vi "live view D06.vi"() -> ()   [LabVIEW 2019, in "D06.lvlib"]
uses:
  D06.lvlib
  <vilib>/userDefined/High Color/IMAQdx.ctl
  <vilib>/vision/Image Controls.llb/IMAQ Image.ctl
  <vilib>/measure/mamon.llb/Trigger Detection for 1 Channel.vi
  <vilib>/measure/NI_MAPro.lvlib
  Calibration Lib.lvlib
  database.lvlib
  <vilib>/vision/driver/NI_Vision_Acquisition_Software.lvlib
panel:
  out "error out":errorcluster
  in  "snapshot":bool
  out "projector D06 error":errorcluster
  in  "Path":path
  in  "Verify Calibration D06":bool caption="capture grab"
  out "factor":sgl
  out "transform matrix":sgl[](array[numeric])
  in  "Method 2 save D06":bool caption="capture grab"
  in  "Method 1 Save D06":bool caption="Saving txt"
  in  "Close":bool
  out "Average Result":string="Average Result"
  out ">18  A":dbl(slide)=1.0 caption=">18 mm" scale=0.0..100.0
  out "16-18  A":dbl(slide)=1.0 caption="16-18 mm" scale=0.0..100.0
  out "14-16  A":dbl(slide)=1.0 caption="14-16 mm" scale=0.0..100.0
  out "12.5-14 A":dbl(slide)=1.0 caption="12.5-14 mm" scale=0.0..100.0
  out "10-12.5  A":dbl(slide)=1.0 caption="10-12.5 mm" scale=0.0..100.0 scale format="%#_4f"
  out "8-10  A":dbl(slide)=1.0 caption="8-10 mm" scale=0.0..100.0
  out "6.3-8  A":dbl(slide)=1.0 caption="6.3-8 mm" scale=0.0..100.0
  out "<6.3  A":dbl(slide)=1.0 caption="<6.3 mm" scale=0.0..100.0
  out "Live Result":string="Live Result"
  out ">18  L":dbl(slide)=1.0 caption=">18 mm" scale=0.0..100.0
  out "Live View":T1(plugin-control) caption="Disc 26"
  out "16-18  L":dbl(slide)=1.0 caption="16-18 mm" scale=0.0..100.0
  out "14-16  L":dbl(slide)=1.0 caption="14-16 mm" scale=0.0..100.0
  out "12.5-14 L":dbl(slide)=1.0 caption="12.5-14 mm" scale=0.0..100.0
  out "10-12.5  L":dbl(slide)=1.0 caption="10-12.5 mm" scale=0.0..100.0 scale format="%#_4f"
  out "8-10  L":dbl(slide)=1.0 caption="8-10 mm" scale=0.0..100.0
  out "6.3-8  L":dbl(slide)=1.0 caption="6.3-8 mm" scale=0.0..100.0
  out "<6.3  L":dbl(slide)=1.0 caption="<6.3 mm" scale=0.0..100.0
  out "disc name":string="Live Info Disc 06"
  out "dsgs":string="DSGS"
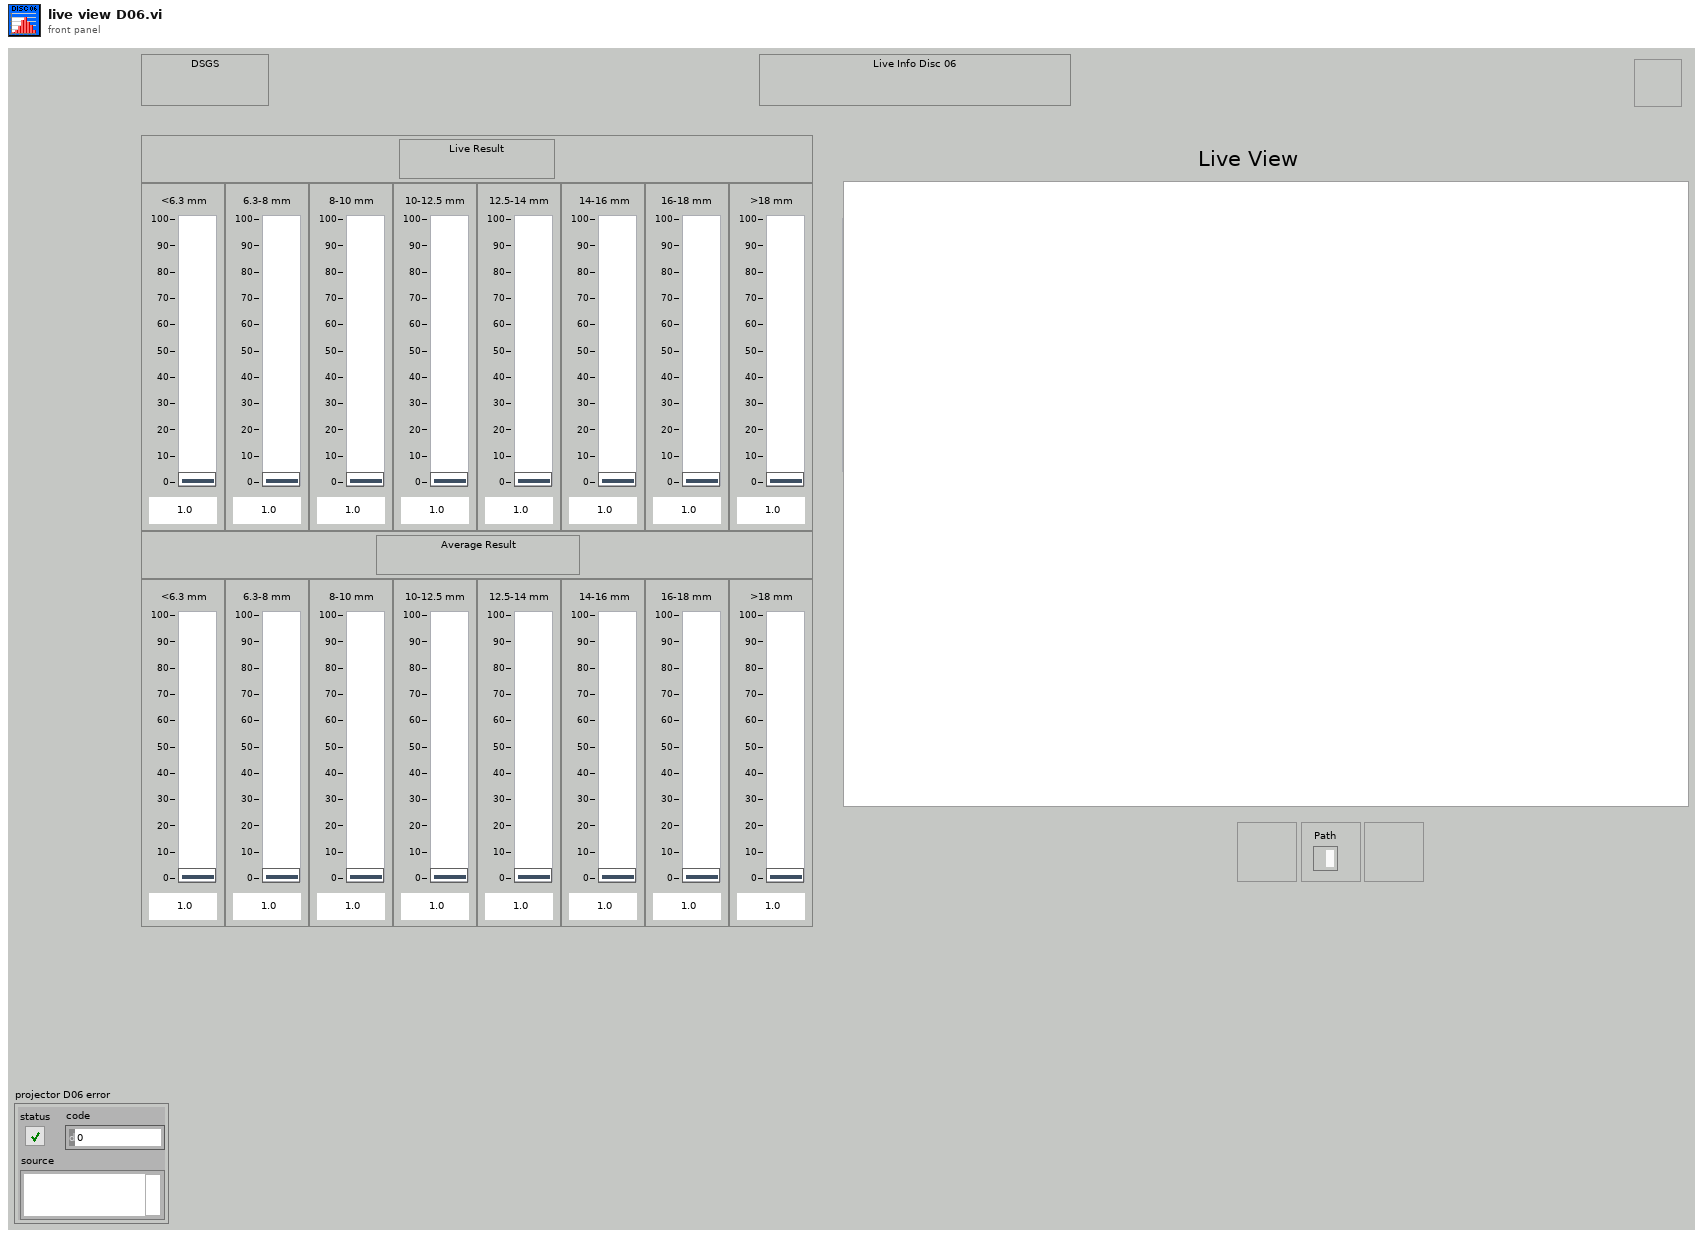
[diagram p1: front panel]
types:
  T1 = typedef "IMAQ Image.ctl" = refnum<image>
  T2 = typedef "Image Type" = u32
  T3 = typedef "IMAQdx.ctl" = refnum<k21>
  T4 = enum8{"Enabled", "Disabled", "Disabled and Grayed Out"}
  T5 = cluster{"date/time string":string, "date/time string":string, "date/time string":string, string, "spreadsheet string":string, string}
  T6 = cluster{"date/time string":string, "date/time string":string, string, "Value":dbl, "Value":dbl, "Value":dbl, "Value":dbl, "Value":dbl, "Value":dbl, "Value":dbl, "Value":dbl}
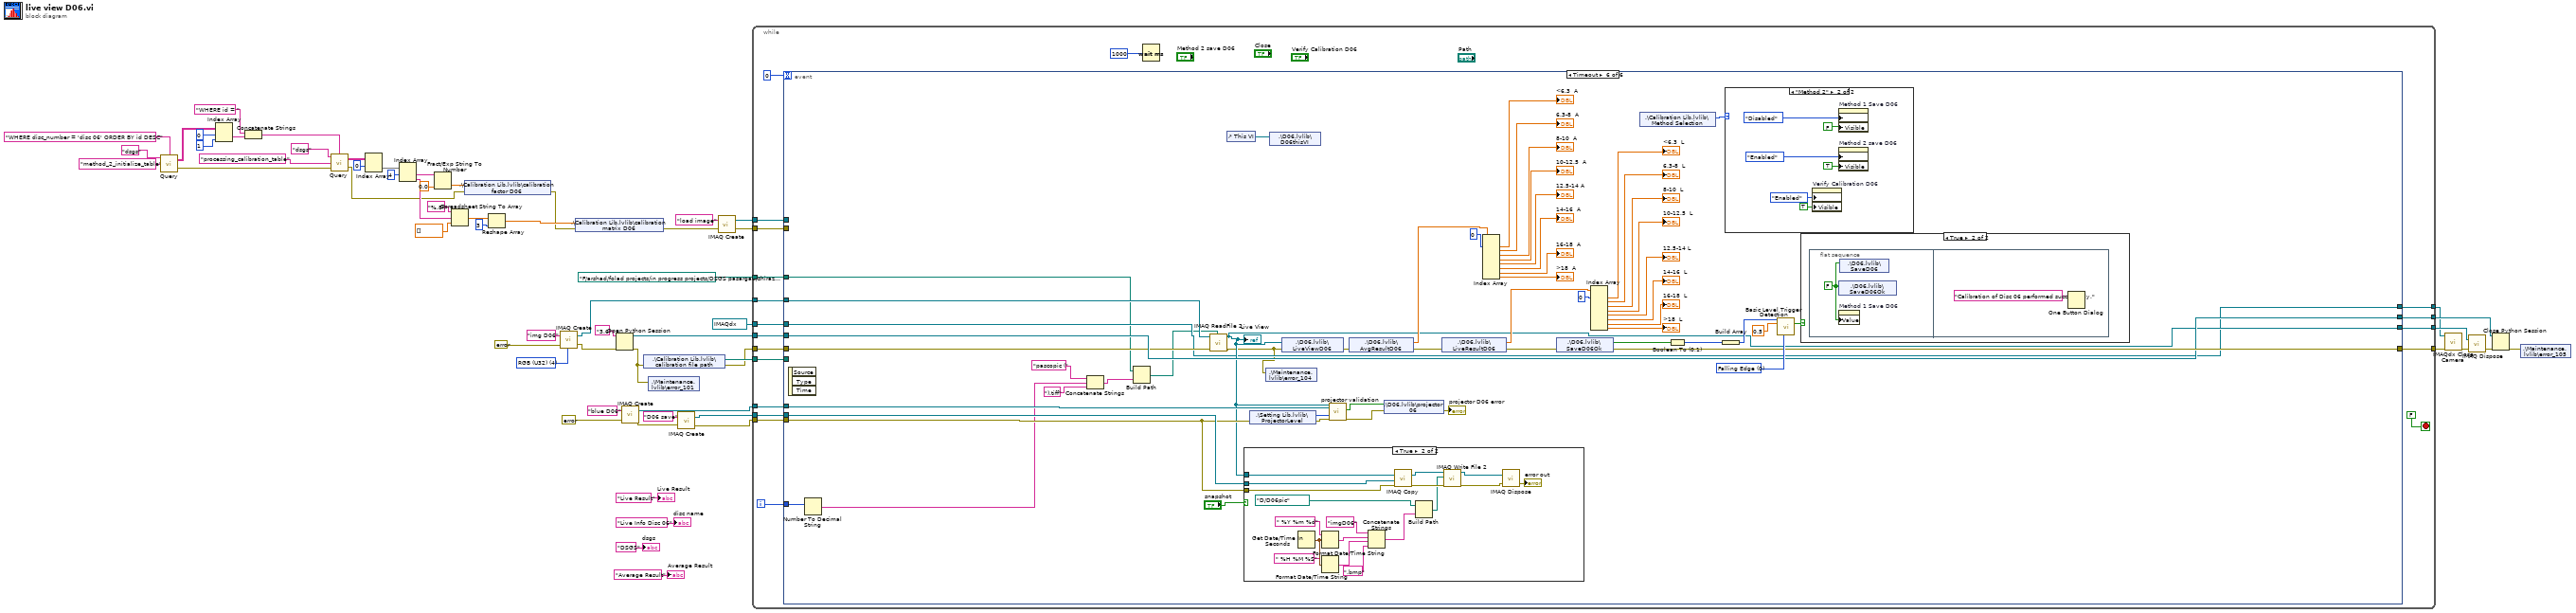
[diagram p0: block diagram]
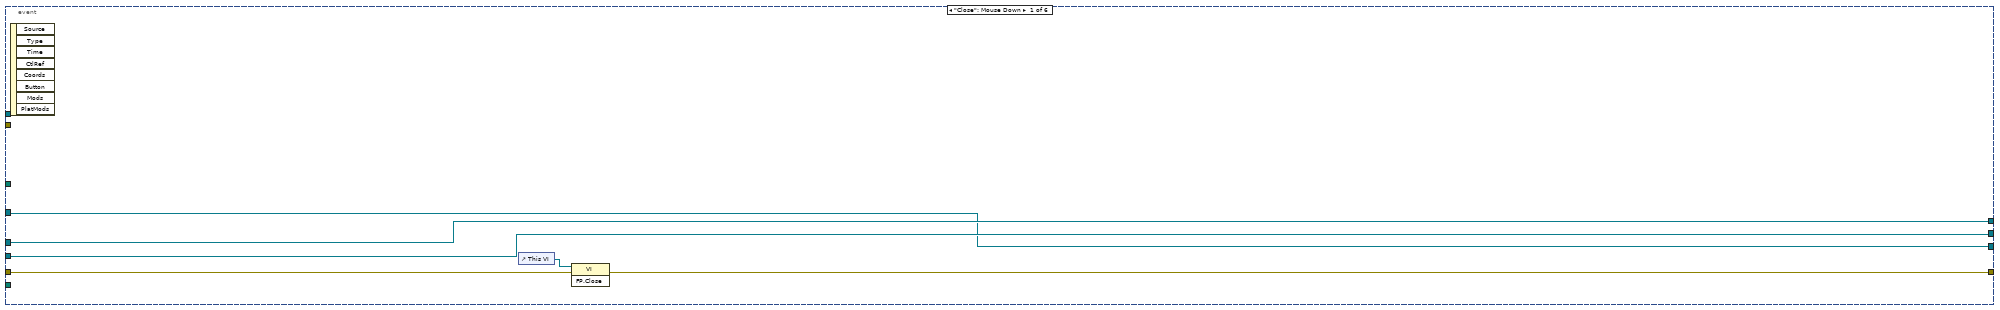
[diagram p2: hidden frame]
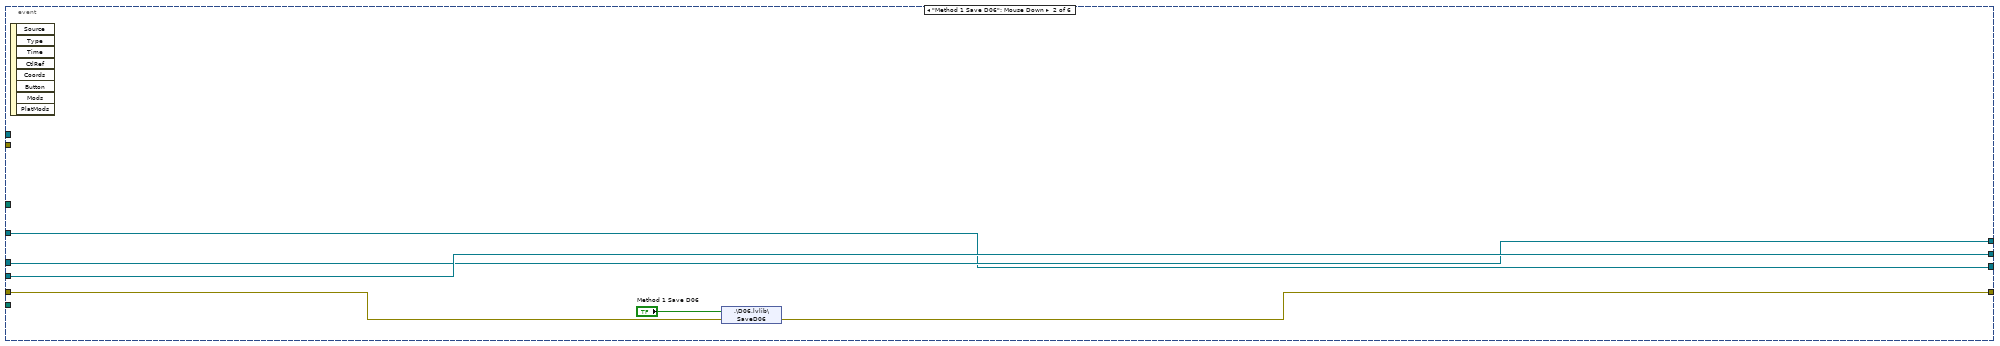
[diagram p3: hidden frame]
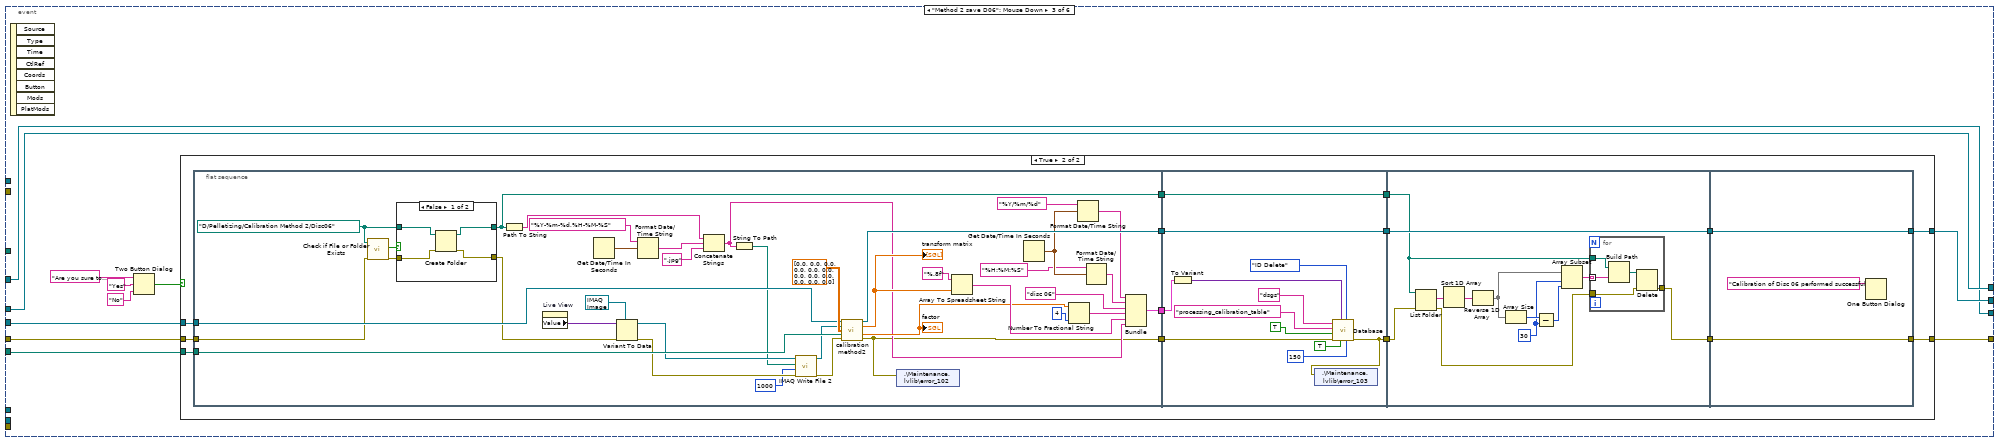
[diagram p4: hidden frame]
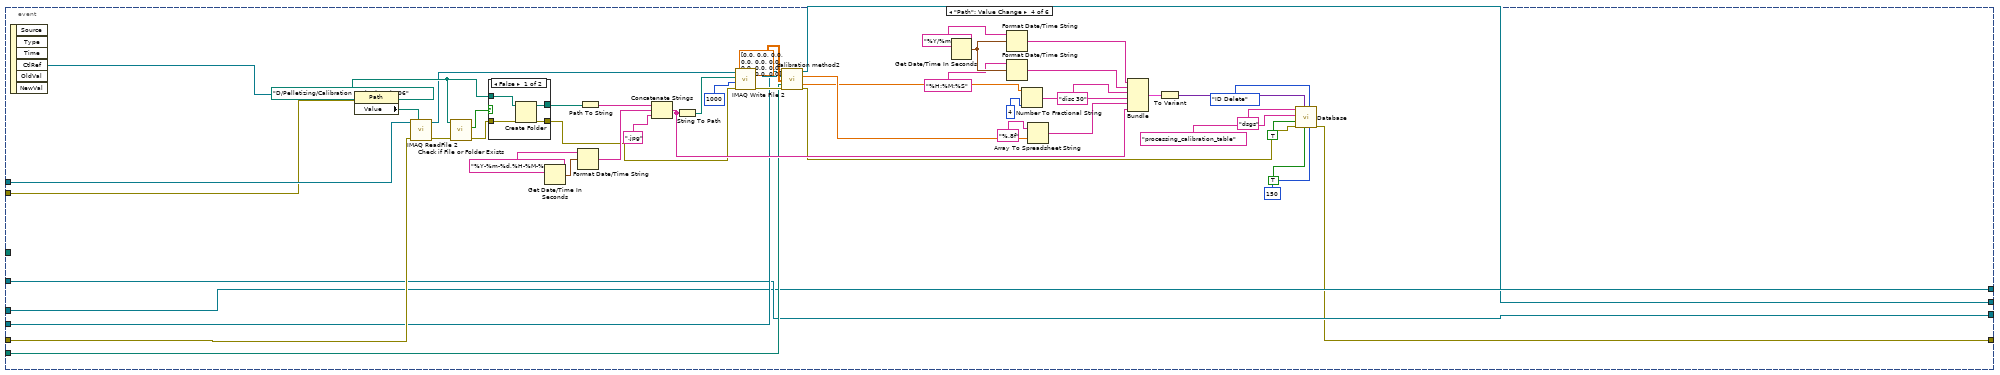
[diagram p7: hidden frame]
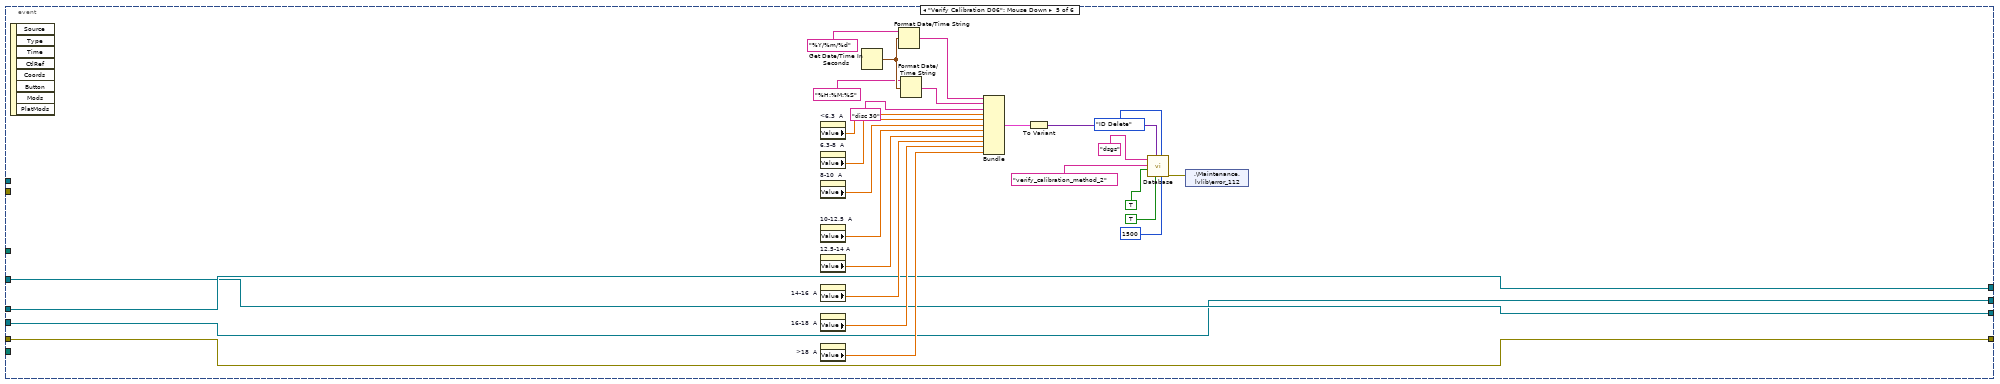
[diagram p9: hidden frame]
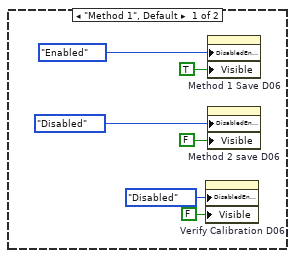
[diagram p11: hidden frame]
diagram:
  w5 = T2 4 items=["Grayscale (U8)", "Grayscale (I16)", "Grayscale (SGL)", "Complex (CSG)", "RGB (U32)", "HSL (U32)", "RGB (U64)", "Grayscale (U16)"] ("Image Type")
  n1 = call "Query.vi"("Condition"="WHERE disc_number = 'disc 06' ORDER BY id DESC", "Table Name"="method_2_initialize_table", "Connection Name"="dsgs") -> ("Error out"=w33:errorcluster, "data"=w38:string[][])  [unwired: 1 in]
  n2 = Index Array(array=w38, index (row)=0, index (col)=1 ("disabled index (col)")) -> (element=w31:string)
  n3 = Concatenate Strings("WHERE id = " ("string"), w31) -> (w30:string)
  n4 = call "Query.vi"("Condition"=w30, "Error in"=w33, "Table Name"="processing_calibration_table", "Connection Name"="dsgs") -> ("Error out"=w15:errorcluster, "data"=w29:string[][])
  n5 = Index Array(array=w29, index (row)=0) -> (element=w27:string[])  [unwired: 1 in]
  n6 = Index Array(array=w27, index #1=4 ("index")) -> (element #1=w25:string, element #2=w18:string)  [unwired: 1 in]
  n7 = Fract/Exp String To Number(string=w25, default (0 dbl)=sgl 0.0 ("default (0 DBL)")) -> (number=w24:sgl)  [unwired: 2 in, 1 out]
  n8 = Spreadsheet String To Array(format string="%.8f", spreadsheet string=w18, array type (2D Dbl)=sgl[] []) -> (array=w21:sgl[])  [unwired: 1 in]
  n9 = shared-variable ".\\Calibration Lib.lvlib\\calibration factor D06"(w24, error in=w15) -> (error out=w16:errorcluster)
  n10 = Reshape Array(w21, 3 ("dimension size")) -> (w17:sgl[])
  n11 = call "IMAQ Create"("Image Name"="img D06", "Image Type"=w5, "error in (no error)"=errorcluster {"status"=FALSE, "code"=0, "source"=""}) -> ("New Image"=w3:T1, "error out"=w2:errorcluster)  [unwired: 2 in]
  n12 = shared-variable ".\\Calibration Lib.lvlib\\calibration matrix D06"(w17, error in=w16) -> (error out=w14:errorcluster)
  n13 = Open Python Session(python version="3.6" ("Python version"), 3:w2) -> (session out=w56:refnum<k35>, error out=w45:errorcluster)  [unwired: 1 in]
  n14 = call "IMAQ Create"("Image Name"="blue D06", "error in (no error)"=errorcluster {"status"=FALSE, "code"=0, "source"=""}) -> ("New Image"=w11:T1, "error out"=w10:errorcluster)  [unwired: 3 in]
  n15 = shared-variable ".\\Calibration Lib.lvlib\\calibration file path"(error in=w45) -> (w48:path, error out=w47:errorcluster)
  n16 = shared-variable ".\\Maintenance.lvlib\\error_101"(w45) -> ()  [unwired: 1 in, 1 out]
  n17 = call "IMAQ Create"("Image Name"="D06 save", "error in (no error)"=w10) -> ("New Image"=w7:T1, "error out"=w9:errorcluster)  [unwired: 3 in]
  n18 = call "IMAQ Create"("Image Name"="load image", "error in (no error)"=w14) -> ("New Image"=w44:T1, "error out"=w43:errorcluster)  [unwired: 3 in]
  n19 = while {
    tunnel: w56 -> [w78]
    tunnel: w48 -> [w77]
    tunnel: w47 -> [w76]
    tunnel: w3 -> [w74]
    tunnel: [w73] -> w55
    tunnel: [w72] -> w52
    tunnel: [w71] -> w54
    tunnel: T3 "disc06" ("Session In") -> [w70]
    tunnel: [w69] -> w49
    tunnel: w44 -> [w68]
    tunnel: w43 -> [w67]
    tunnel: w11 -> [w66]
    tunnel: w9 -> [w65]
    tunnel: w7 -> [w64]
    tunnel: path "F:/arshad/folad projects/in progress projects/DSGS pasargad/shiraz pics" ("base path") -> [w62]
    i -> [w63]
    stop <- FALSE stop-if-true
    n20 = event shown="[5] Timeout" {
      selector: _ -> [_ _ _ _ _ _]
      dyn-events: _ -> [_ _ _ _ _ _]
      timeout: 0 -> [_ _ _ _ _ _]
      tunnel: w78 -> [w84 w90 w103 w200 w254 w300]
      tunnel: w77 -> [_ _ w102 w201 _ _]
      tunnel: [w86 w92 w97 w197 w257 w303] -> w72
      tunnel: w76 -> [w85 w91 w101 w202 w257 w286]
      tunnel: w74 -> [w81 w88 w98 w199 w255 w285]
      tunnel: [w81 w88 w98 w199 w255 w284] -> w73
      tunnel: [w84 w90 w100 w196 w254 w300] -> w71
      tunnel: w70 -> [w82 w89 w99 w198 w256 w283]
      tunnel: [w82 w89 w99 w198 w256 w283] -> w69
      tunnel: w68 -> [_ _ _ w204 _ _]
      tunnel: w67 -> [_ _ _ w203 _ _]
      tunnel: w66 -> [_ _ _ _ _ w294]
      tunnel: w65 -> [_ _ _ _ _ w291]
      tunnel: w64 -> [_ _ _ _ _ w292]
      tunnel: w63 -> [_ _ _ _ _ w287]
      tunnel: w62 -> [_ _ _ _ _ w281]
      event "Close": Mouse Down {
        n21 = event-data() -> ()  [unwired: 1 in, 8 out]
        n22 = control-ref of="This VI"() -> (w83:refnum<vi>)
        n23 = invoke class="VI" method="FP.Close"(reference=w83, error in=w85) -> (error out=w86:errorcluster)  [unwired: 1 in, 2 out]
      }
      event "Method 1 Save D06": Mouse Down {
        n24 = event-data() -> ()  [unwired: 1 in, 8 out]
        n25 = shared-variable ".\\D06.lvlib\\SaveD06"("Method 1 Save D06", error in=w91) -> (error out=w92:errorcluster)
      }
      event "Method 2 save D06": Mouse Down {
        n26 = event-data() -> ()  [unwired: 1 in, 8 out]
        n27 = Two Button Dialog(message="Are you sure to calibration Disc 30?", 1:"No" ("F button name (\"Cancel\")"), 2:"Yes" ("T button name (\"OK\")")) -> (T button?=w93:bool)
        n28 = case shown="True" w93 {
          tunnel: w103 -> [w104 w112]
          tunnel: w102 -> [_ w111]
          tunnel: w101 -> [w105 w110]
          tunnel: [w104 w109] -> w100
          tunnel: [w105 w108] -> w97
          frame False {
          }
          frame True {
            n29 = flat-sequence {
              tunnel: [w157] -> w119
              tunnel: [w123] -> w118
              tunnel: [w148] -> w117
              tunnel: w110 -> [w129]
              tunnel: w111 -> [w147]
              tunnel: w112 -> [w139]
              tunnel: [w122] -> w116
              tunnel: w119 -> [w175]
              tunnel: w118 -> [w173]
              tunnel: w117 -> [w168]
              tunnel: [w175] -> w115
              tunnel: [w169] -> w114
              tunnel: [w166] -> w113
              tunnel: w116 -> [w166]
              tunnel: w115 -> [w187]
              tunnel: w114 -> [w177]
              tunnel: w113 -> [w176]
              tunnel: [w187] -> w107
              tunnel: [w178] -> w106
              tunnel: [w194] -> w108
              tunnel: [w195] -> w109
              tunnel: w107 -> [w195]
              tunnel: w106 -> [w194]
              frame #0 {
                w133 = path "D:/Pelletizing/Calibration Method 2/Disc06" ("path")
                n30 = call <vilib>:"Check if File or Folder Exists.vi"("error in (no error)"=w129, "path"=w133) -> ("error out"=w131:errorcluster, "file or folder exists?"=w134:bool)  [unwired: 7 in, 1 out]
                n31 = case shown="False" w134 {
                  tunnel: [w159 w163] -> w122
                  tunnel: w133 -> [w161 w163]
                  tunnel: w131 -> [w160 w162]
                  tunnel: [w158 w162] -> w128
                  frame False {
                    n32 = Create Folder(path (use dialog)=w161, error in=w160) -> (created path=w159:path, error out=w158:errorcluster)  [unwired: 1 in, 1 out]
                  }
                  frame True {
                  }
                }
                n33 = Path To String(path=w122) -> (string=w132:string)
                n34 = property on="Live View" class="ImageControl"() -> ("Value"=w146:variant)  [unwired: 2 in, 2 out]
                n35 = Get Date/Time In Seconds() -> (seconds since 1Jan1904=w138:timestamp)
                n36 = Variant To Data(error in=w128, type=T1 refnum ("New Image"), Variant=w146) -> (data=w127:T1, error out=w126:errorcluster)
                n37 = Format Date/Time String(time format string (%c)="%Y-%m-%d,%H-%M-%S", seconds (now)=w138) -> (date/time string=w136:string)  [unwired: 1 in]
                n38 = Concatenate Strings(w132, w136, ".jpg" ("string")) -> (w130:string)
                n39 = String To Path(string=w130) -> (path=w125:path)
                n40 = call-poly "IMAQ Write File 2"("error in (no error)"=w126, "Image Quality"=u32 1000, "File Path"=w125, "Image"=w127) -> ("error out"=w120:errorcluster, "Image Out (duplicate)"=w121:T1)  [unwired: 6 in]
                n41 = call "calibration method2.vi"("session in"=w139, "Image IN"=w121, "initialize matrix"=sgl[][] [[0.0, 0.0, 0.0], [0.0, 0.0, 0.0], [0.0, 0.0, 0.0], [0.0, 0.0, 0.0]] ("(4*3) array"), "module path"=w147, "error in"=w120) -> ("session out"=w157:refnum<k35>, "calibration vector"=w141:sgl[], "factor"=w143:sgl, "error out"=w123:errorcluster)  [unwired: 6 in, 1 out]
                "factor" <- w143
                "transform matrix" <- w141
                n42 = shared-variable ".\\Maintenance.lvlib\\error_102"(w123) -> ()  [unwired: 1 in, 1 out]
                n43 = Array To Spreadsheet String(array=w141, 3:"%.8f" ("format string")) -> (spreadsheet string=w149:string)  [unwired: 1 in]
                n44 = Get Date/Time In Seconds() -> (seconds since 1Jan1904=w154:timestamp)
                n45 = Number To Fractional String(number=w143, precision (6)=i16 4) -> (F-format string=w150:string)  [unwired: 2 in]
                n46 = Format Date/Time String(time format string (%c)="%Y/%m/%d", seconds (now)=w154) -> (date/time string=w155:string)  [unwired: 1 in]
                n47 = Format Date/Time String(time format string (%c)="%H:%M:%S", seconds (now)=w154) -> (date/time string=w156:string)  [unwired: 1 in]
                n48 = Bundle("date/time string"=w155, "date/time string"=w156, "date/time string"="disc 06", w150, "spreadsheet string"=w149, w130) -> (w148:T5)  [unwired: 1 in]
              }
              frame #1 {
                n49 = To Variant(anything=w168) -> (Variant=w167:variant)
                n50 = call "Database.vi"("Maximum Row"=150, "Enum"=enum16{"ID Delete", "Time Delete"}."ID Delete", "Delete row?"=TRUE, "Data"=w167, "Error in"=w173, "Auto Increment ID?"=TRUE, "Table"="processing_calibration_table", "Connection"="dsgs") -> ("Error out"=w169:errorcluster)  [unwired: 3 in]
                n51 = shared-variable ".\\Maintenance.lvlib\\error_103"(w169) -> ()  [unwired: 1 in, 1 out]
              }
              frame #2 {
                w180 = 30 ("index")
                n52 = List Folder(path=w176, error in=w177) -> (filenames=w181:string[], error out=w179:errorcluster)  [unwired: 2 in, 2 out]
                n53 = Sort 1D Array(array=w181) -> (sorted array=w182:string[])
                n54 = Reverse 1D Array(array=w182) -> (reversed array=w183:string[])
                n55 = Array Size(array=w183) -> (size(s)=w184:i32)
                n56 = Subtract(x=w184, y=w180) -> (x-y=w185:i32)
                n57 = Array Subset(array=w183, index=w180, length=w185) -> (w186:string[])
                n58 = for {
                  tunnel: w186 -> [w191] mode=indexing
                  tunnel: w176 -> [w192]
                  tunnel: [w189] -> w178
                  tunnel: w179 -> [w188]
                  n59 = Build Path(base path=w192, name or relative path=w191) -> (appended path=w190:path)
                  n60 = Delete(path (use dialog)=w190, error in=w188) -> (error out=w189:errorcluster)  [unwired: 3 in, 2 out]
                }
              }
              frame #3 {
                n61 = One Button Dialog(message="Calibration of Disc 06 performed successfully.") -> ()  [unwired: 1 in, 1 out]
              }
            }
          }
        }
      }
      event "Path": Value Change {
        w237 = path "D:/Pelletizing/Calibration Method 2/Disc06" ("path")
        n62 = event-data() -> ("CtlRef"=w205:refnum<vi>)  [unwired: 1 in, 5 out]
        n63 = property class="Path"(reference=w205, error in=w203) -> ("Value"=w232:path)  [unwired: 2 out]
        n64 = call "IMAQ ReadFile 2"("File Path"=w232, "error in (no error)"=w202, "Image"=w204) -> ("error out"=w230:errorcluster, "Image Out"=w231:T1)  [unwired: 4 in, 3 out]
        n65 = call <vilib>:"Check if File or Folder Exists.vi"("error in (no error)"=w230, "path"=w237) -> ("error out"=w234:errorcluster, "file or folder exists?"=w238:bool)  [unwired: 7 in, 1 out]
        n66 = case shown="False" w238 {
          tunnel: [w247 w251] -> w236
          tunnel: w237 -> [w249 w251]
          tunnel: w234 -> [w248 w250]
          tunnel: [w246 w250] -> w207
          frame False {
            n67 = Create Folder(path (use dialog)=w249, error in=w248) -> (created path=w247:path, error out=w246:errorcluster)  [unwired: 1 in, 1 out]
          }
          frame True {
          }
        }
        n68 = Get Date/Time In Seconds() -> (seconds since 1Jan1904=w242:timestamp)
        n69 = Format Date/Time String(time format string (%c)="%Y-%m-%d,%H-%M-%S", seconds (now)=w242) -> (date/time string=w240:string)  [unwired: 1 in]
        n70 = Path To String(path=w236) -> (string=w235:string)
        n71 = Concatenate Strings(w235, w240, ".jpg" ("string")) -> (w218:string)
        n72 = String To Path(string=w218) -> (path=w233:path)
        n73 = call-poly "IMAQ Write File 2"("error in (no error)"=w207, "Image Quality"=u32 1000, "File Path"=w233, "Image"=w231) -> ("error out"=w244:errorcluster, "Image Out (duplicate)"=w229:T1)  [unwired: 6 in]
        n74 = call "calibration method2.vi"("session in"=w200, "Image IN"=w229, "initialize matrix"=sgl[][] [[0.0, 0.0, 0.0], [0.0, 0.0, 0.0], [0.0, 0.0, 0.0], [0.0, 0.0, 0.0]] ("(4*3) array"), "module path"=w201, "error in"=w244) -> ("session out"=w196:refnum<k35>, "calibration vector"=w217:sgl[], "factor"=w216:sgl, "error out"=w206:errorcluster)  [unwired: 6 in, 1 out]
        n75 = Get Date/Time In Seconds() -> (seconds since 1Jan1904=w226:timestamp)
        n76 = Format Date/Time String(time format string (%c)="%Y/%m/%d", seconds (now)=w226) -> (date/time string=w227:string)  [unwired: 1 in]
        n77 = Format Date/Time String(time format string (%c)="%H:%M:%S", seconds (now)=w226) -> (date/time string=w228:string)  [unwired: 1 in]
        n78 = Number To Fractional String(number=w216, precision (6)=i16 4) -> (F-format string=w222:string)  [unwired: 2 in]
        n79 = Array To Spreadsheet String(array=w217, 3:"%.8f" ("format string")) -> (spreadsheet string=w221:string)  [unwired: 1 in]
        n80 = Bundle("date/time string"=w227, "date/time string"=w228, "date/time string"="disc 30", w222, "spreadsheet string"=w221, w218) -> (w208:T5)  [unwired: 1 in]
        n81 = To Variant(anything=w208) -> (Variant=w211:variant)
        n82 = call "Database.vi"("Maximum Row"=150, "Enum"=enum16{"ID Delete", "Time Delete"}."ID Delete", "Delete row?"=TRUE, "Data"=w211, "Error in"=w206, "Auto Increment ID?"=TRUE, "Table"="processing_calibration_table", "Connection"="dsgs") -> ("Error out"=w197:errorcluster)  [unwired: 3 in]
      }
      event "Verify Calibration D06": Mouse Down {
        n83 = event-data() -> ()  [unwired: 1 in, 8 out]
        n84 = property on="<6.3  A" class="Slide (strict)"() -> ("Value"=w275:dbl)  [unwired: 2 in, 2 out]
        n85 = property on="6.3-8  A" class="Slide (strict)"() -> ("Value"=w274:dbl)  [unwired: 2 in, 2 out]
        n86 = property on="8-10  A" class="Slide (strict)"() -> ("Value"=w273:dbl)  [unwired: 2 in, 2 out]
        n87 = property on="10-12.5  A" class="Slide (strict)"() -> ("Value"=w272:dbl)  [unwired: 2 in, 2 out]
        n88 = property on="12.5-14 A" class="Slide (strict)"() -> ("Value"=w271:dbl)  [unwired: 2 in, 2 out]
        n89 = property on="14-16  A" class="Slide (strict)"() -> ("Value"=w270:dbl)  [unwired: 2 in, 2 out]
        n90 = property on="16-18  A" class="Slide (strict)"() -> ("Value"=w269:dbl)  [unwired: 2 in, 2 out]
        n91 = property on=">18  A" class="Slide (strict)"() -> ("Value"=w268:dbl)  [unwired: 2 in, 2 out]
        n92 = Get Date/Time In Seconds() -> (seconds since 1Jan1904=w278:timestamp)
        n93 = Format Date/Time String(time format string (%c)="%Y/%m/%d", seconds (now)=w278) -> (date/time string=w277:string)  [unwired: 1 in]
        n94 = Format Date/Time String(time format string (%c)="%H:%M:%S", seconds (now)=w278) -> (date/time string=w276:string)  [unwired: 1 in]
        n95 = Bundle("date/time string"=w277, "date/time string"=w276, "disc 30", "Value"=w275, "Value"=w274, "Value"=w273, "Value"=w272, "Value"=w271, "Value"=w270, "Value"=w269, "Value"=w268) -> (w267:T6)  [unwired: 1 in]
        n96 = To Variant(anything=w267) -> (Variant=w266:variant)
        n97 = call "Database.vi"("Maximum Row"=1500, "Enum"=enum16{"ID Delete", "Time Delete"}."ID Delete", "Delete row?"=TRUE, "Data"=w266, "Auto Increment ID?"=TRUE, "Table"="verify_calibration_method_2", "Connection"="dsgs") -> ("Error out"=w265:errorcluster)  [unwired: 4 in]
        n98 = shared-variable ".\\Maintenance.lvlib\\error_112"(w265) -> ()  [unwired: 1 in, 1 out]
      }
      event Timeout {
        w308 = u16 0 items=["Falling Edge", "Rising Edge"] ("trigger slope")
        n99 = event-data() -> ()  [unwired: 1 in, 3 out]
        n100 = Number To Decimal String(number=w287) -> (decimal integer string=w280:string)  [unwired: 1 in]
        n101 = Concatenate Strings("pascopic (" ("string"), w280, ").tiff" ("string")) -> (w290:string)
        n102 = Build Path(base path=w281, name or relative path=w290) -> (appended path=w279:path)
        n103 = call "IMAQ ReadFile 2"("File Path"=w279, "error in (no error)"=w286, "Image"=w285) -> ("error out"=w282:errorcluster, "Image Out"=w284:T1)  [unwired: 4 in, 3 out]
        "Live View" <- w284
        n104 = control-ref of="This VI"() -> (w301:refnum<vi>)
        n105 = case shown="True" "snapshot" {
          tunnel: w292 -> [_ w350]
          tunnel: w284 -> [_ w349]
          tunnel: w291 -> [_ w333]
          frame False {
          }
          frame True {
            n106 = Get Date/Time In Seconds() -> (seconds since 1Jan1904=w343:timestamp)
            n107 = Format Date/Time String(time format string (%c)=" %Y %m %d", seconds (now)=w343) -> (date/time string=w339:string)  [unwired: 1 in]
            n108 = Format Date/Time String(time format string (%c)=" %H %M %S", seconds (now)=w343) -> (date/time string=w338:string)  [unwired: 1 in]
            n109 = Concatenate Strings("imgD06" ("string"), w339, w338, ".bmp" ("string")) -> (w336:string)
            n110 = call "IMAQ Copy"("error in (no error)"=w333, "Image Dst"=w350, "Image Src"=w349) -> ("error out"=w347:errorcluster, "Image Dst Out"=w348:T1)  [unwired: 3 in]
            n111 = Build Path(base path=path "D:/D06pic" ("File Path"), name or relative path=w336) -> (appended path=w335:path)
            n112 = call-poly "IMAQ Write File 2"("error in (no error)"=w347, "File Path"=w335, "Image"=w348) -> ("error out"=w345:errorcluster, "Image Out (duplicate)"=w346:T1)  [unwired: 7 in]
            n113 = call "IMAQ Dispose"("Image"=w346, "error in (no error)"=w345) -> ("error out"=→"error out":errorcluster)  [unwired: 4 in]
          }
        }
        n114 = shared-variable ".\\Setting Lib.lvlib\\ProjectorLevel"(error in=w291) -> (w299:i32, error out=w298:errorcluster)
        n115 = shared-variable ".\\Maintenance.lvlib\\error_104"(w282) -> ()  [unwired: 1 in, 1 out]
        n116 = shared-variable ".\\D06.lvlib\\D06thisVI"(w301) -> ()  [unwired: 1 in, 1 out]
        n117 = shared-variable ".\\D06.lvlib\\LiveViewD06"(w284, error in=w282) -> (error out=w302:errorcluster)
        n118 = call "projector validation.vi"("Image Src"=w284, "blue channel"=w294, "on/off level"=w299, "error in (no error)"=w298) -> ("on/off"=w297:bool, "error out"=w296:errorcluster)  [unwired: 14 in]
        n119 = shared-variable ".\\D06.lvlib\\AvgResultD06"(error in=w302) -> (w323:dbl[], error out=w305:errorcluster)
        n120 = shared-variable ".\\D06.lvlib\\projector 06"(w297, error in=w296) -> (error out=→"projector D06 error":errorcluster)
        n121 = shared-variable ".\\D06.lvlib\\LiveResultD06"(error in=w305) -> (w322:dbl[], error out=w304:errorcluster)
        n122 = Index Array(array=w323, index #1=0 ("index")) -> (element #1=→"<6.3  A":dbl, element #2=→"6.3-8  A":dbl, element #3=→"8-10  A":dbl, element #4=→"10-12.5  A":dbl, element #5=→"12.5-14 A":dbl, element #6=→"14-16  A":dbl, element #7=→"16-18  A":dbl, element #8=→">18  A":dbl)  [unwired: 7 in]
        n123 = shared-variable ".\\D06.lvlib\\SaveD06Ok"(error in=w304) -> (w309:bool, error out=w303:errorcluster)
        n124 = Index Array(array=w322, index #1=0 ("index")) -> (element #1=→"<6.3  L":dbl, element #2=→"6.3-8  L":dbl, element #3=→"8-10  L":dbl, element #4=→"10-12.5  L":dbl, element #5=→"12.5-14 L":dbl, element #6=→"14-16  L":dbl, element #7=→"16-18  L":dbl, element #8=→">18  L":dbl)  [unwired: 7 in]
        n125 = shared-variable ".\\Calibration Lib.lvlib\\Method Selection"() -> (w306:enum32{"Method 1", "Method 2"})  [unwired: 1 in, 1 out]
        n126 = Boolean To (0,1)(Boolean=w309) -> (0, 1=w312:i16)
        n127 = Build Array(w312) -> (w311:i16[])
        n128 = case shown="\"Method 2\"" w306 {
          frame "Method 1", Default {
            n129 = property on="Verify Calibration D06" class="Bool (strict)"("DisabledEnum"=T4."Disabled" ("Disabled"), "Visible"=FALSE) -> ()  [unwired: 2 in, 2 out]
            n130 = property on="Method 1 Save D06" class="Bool (strict)"("DisabledEnum"=T4."Enabled" ("Disabled"), "Visible"=TRUE) -> ()  [unwired: 2 in, 2 out]
            n131 = property on="Method 2 save D06" class="Bool (strict)"("DisabledEnum"=T4."Disabled" ("Disabled"), "Visible"=FALSE) -> ()  [unwired: 2 in, 2 out]
          }
          frame "Method 2" {
            n132 = property on="Verify Calibration D06" class="Bool (strict)"("DisabledEnum"=T4."Enabled" ("Disabled"), "Visible"=TRUE) -> ()  [unwired: 2 in, 2 out]
            n133 = property on="Method 1 Save D06" class="Bool (strict)"("DisabledEnum"=T4."Disabled" ("Disabled"), "Visible"=FALSE) -> ()  [unwired: 2 in, 2 out]
            n134 = property on="Method 2 save D06" class="Bool (strict)"("DisabledEnum"=T4."Enabled" ("Disabled"), "Visible"=TRUE) -> ()  [unwired: 2 in, 2 out]
          }
        }
        n135 = call-poly <vilib>:"Basic Level Trigger Detection.vi"("signal in"=w311, "level"=0.5, "trigger slope"=w308) -> ("trigger detected?"=w307:bool)  [unwired: 10 in, 2 out]
        n136 = case shown="True" w307 {
          frame False {
          }
          frame True {
            n137 = flat-sequence {
              frame #0 {
                w363 = FALSE
                n138 = shared-variable ".\\D06.lvlib\\SaveD06Ok"(w363) -> ()  [unwired: 1 in, 1 out]
                n139 = property on="Method 1 Save D06" class="Bool (strict)"("Value"=w363) -> ()  [unwired: 2 in, 2 out]
                n140 = shared-variable ".\\D06.lvlib\\SaveD06"(w363) -> ()  [unwired: 1 in, 1 out]
              }
              frame #1 {
                n141 = One Button Dialog(message="Calibration of Disc 06 performed successfully.") -> ()  [unwired: 1 in, 1 out]
              }
            }
          }
        }
      }
    }
    n142 = Wait (ms)(milliseconds to wait=u32 1000) -> ()  [unwired: 1 out]
  }
  n143 = call <vilib>:"IMAQdx Close Camera.vi"("error in"=w52, "Session In"=w49) -> ("error out"=w51:errorcluster)  [unwired: 9 in]
  n144 = call "IMAQ Dispose"("Image"=w55, "error in (no error)"=w51) -> ("error out"=w53:errorcluster)  [unwired: 4 in]
  n145 = Close Python Session(session in=w54, error in=w53) -> (11:w46:errorcluster)
  n146 = shared-variable ".\\Maintenance.lvlib\\error_105"(w46) -> ()  [unwired: 1 in, 1 out]
  "Live Result" <- "Live Result" ("Live Result")
  "Average Result" <- "Average Result" ("Average Result")
  "disc name" <- "Live Info Disc 06" ("Live Result")
  "dsgs" <- "DSGS" ("Live Result")
